vi "MCL Device Attached.vi"(8 "error in (no error)":errorcluster, 10 "handle":i32, 11 "milliseconds":i32) -> (0 "error out":errorcluster, 3 "function return":bool)   [LabVIEW 2014, in "Madlib.lvlib"]
doc: "MADLIB_API bool MCL_DeviceAttached(int milliseconds, int handle);"
uses:
  <userlib>/Lambda2/lib/Madlib/Madlib.lvlib
  <userlib>/Lambda2/lib/Madlib/Madlib.dll
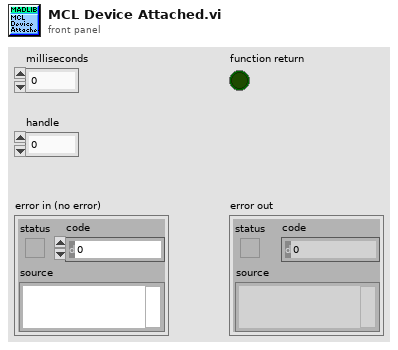
[diagram p1: front panel]
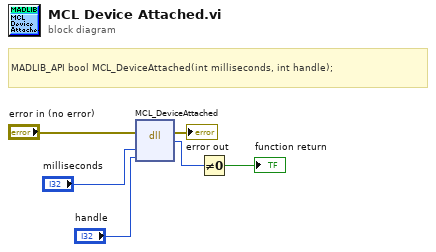
[diagram p0: block diagram]
diagram:
  # "MADLIB_API\tbool\tMCL_DeviceAttached(int milliseconds, int handle);"
  n1 = dll-call lib="C:/Program Files (x86)/National Instruments/LabVIEW 2014/user.lib/Lambda2/lib/Madlib/Madlib.*" fn="MCL_DeviceAttached"(error in="error in (no error)", "milliseconds"="milliseconds", "handle"="handle") -> (error out=→"error out":errorcluster, w5:u8)  [unwired: 4 in, 1 out]
  n2 = Not Equal To 0?(x=w5) -> (x != 0?=→"function return":bool)
